vi "KeithleySendCmd.vi"() -> ()   [LabVIEW 2018]
panel:
  in  "data":string(combo)
  in  "stop":bool
  in  "send":bool
  out "error out":errorcluster
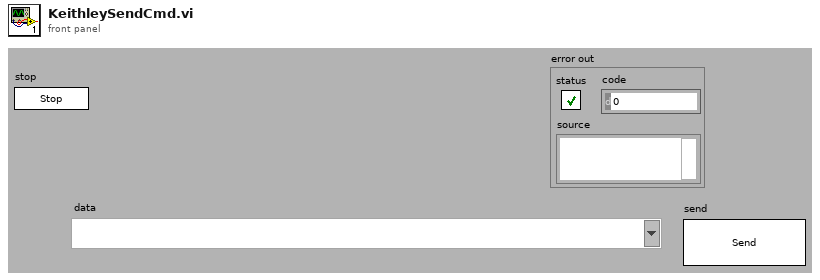
[diagram p1: front panel]
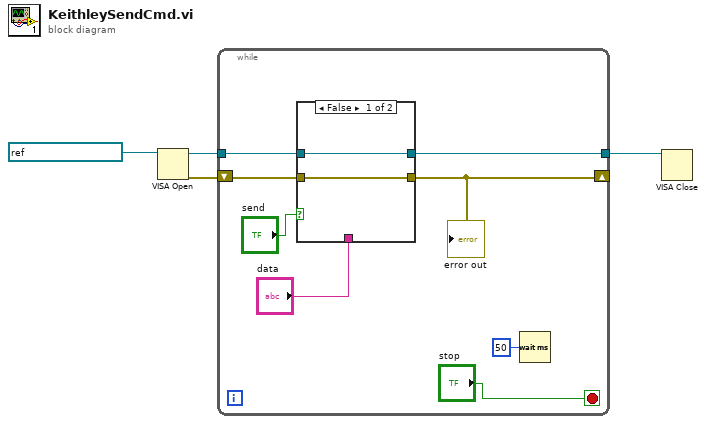
[diagram p0: block diagram]
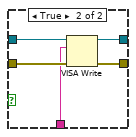
[diagram p2: hidden frame]
diagram:
  n1 = VISA Open(VISA resource name=refnum<visa-resource-name> "GPIB0::24::INSTR") -> (VISA resource name=w2:refnum<visa-resource-name>, error out=w3:errorcluster)  [unwired: 4 in]
  n2 = while {
    tunnel: w2 -> [w11]
    tunnel: [w10] -> w1
    shift-right: [w9] -> _
    shift-left: w3 -> [w12]
    stop <- "stop" stop-if-true
    n3 = case shown="False" "send" {
      tunnel: w12 -> [w13 w19]
      tunnel: w11 -> [w14 w18]
      tunnel: [w14 w17] -> w10
      tunnel: [w13 w16] -> w9
      tunnel: "data" -> [_ w15]
      frame False {
      }
      frame True {
        n4 = VISA Write(VISA resource name=w18, write buffer=w15, error in (no error)=w19) -> (VISA resource name out=w17:refnum<visa-resource-name>, error out=w16:errorcluster)  [unwired: 1 out]
      }
    }
    "error out" <- w9
    n5 = Wait (ms)(milliseconds to wait=u32 50) -> ()  [unwired: 1 out]
  }
  n6 = VISA Close(VISA resource name=w1) -> ()  [unwired: 1 in, 1 out]
